vi "close socket.vi"(8 "error in":errorcluster, 11 "socket":i64) -> (0 "error out":errorcluster)   [LabVIEW 2013, in "lvnano.lvlib"]
doc: "NN_EXPORT int nn_close (int s);"
uses:
  lvnano.lvlib
  lvnanomsg.dll
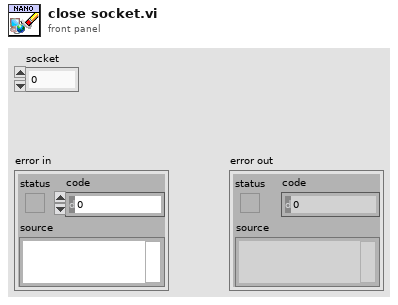
[diagram p1: front panel]
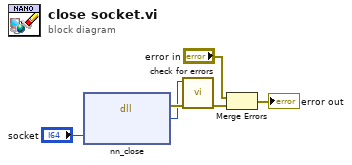
[diagram p0: block diagram]
diagram:
  n1 = dll-call lib="C:/Users/Daniel/Documents/nanomsg/lvnano/lvnanomsg.*" fn="nn_close"("socket"="socket") -> (error out=w5:errorcluster, "error"=w3:i32)  [unwired: 4 in, 1 out]
  n2 = call "check for errors.vi"("error in"=w5, "function return"=w3) -> ("error out"=w4:errorcluster)  [unwired: 9 in]
  n3 = Merge Errors("error in", w4) -> (→"error out":errorcluster)
